vi "Untitled 2.vi"() -> ()   [LabVIEW 2023]
panel:
  out "x-y*floor(x/y) 2":i32
  out "x-y*floor(x/y)":i32
  in  "1":i32
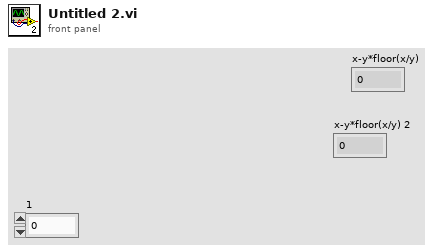
[diagram p1: front panel]
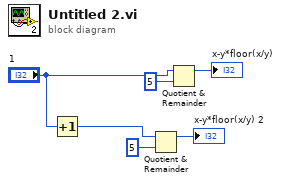
[diagram p0: block diagram]
diagram:
  n1 = Increment(x="1") -> (x+1=w1:i32)
  n2 = Quotient & Remainder(x=w1, y=5) -> (x-y*floor(x/y)=→"x-y*floor(x/y) 2":i32)  [unwired: 1 out]
  n3 = Quotient & Remainder(x="1", y=5) -> (x-y*floor(x/y)=→"x-y*floor(x/y)":i32)  [unwired: 1 out]
